vi "kinectConfigure.vi"(8 "error in (no error)":errorcluster, 10 "Enabled Frames":T2, 11 "KinectSensor References in":T1) -> (0 "error out":errorcluster, 3 "KinectSensor References out":T1)   [LabVIEW 2014]
uses:
  controls/KinectSensor References.ctl
  Microsoft.Kinect
  controls/FrameDescription.ctl
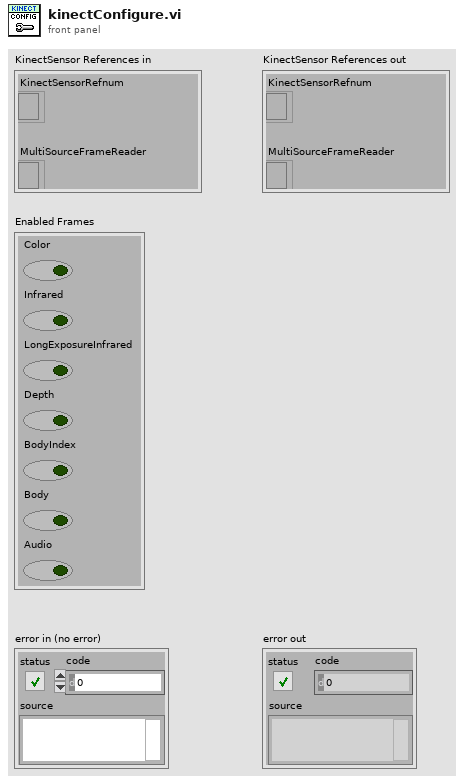
[diagram p1: front panel]
types:
  T1 = typedef "KinectSensor References.ctl" = cluster{"KinectSensorRefnum":refnum<k24>, "MultiSourceFrameReader":refnum<k24>}
  T2 = cluster{"Color":bool, "Infrared":bool, "LongExposureInfrared":bool, "Depth":bool, "BodyIndex":bool, "Body":bool, "Audio":bool}
  T3 = typedef "FrameDescription.ctl" = cluster{"BytesPerPixel":u32, "DiagonalFieldOfView":sgl, "Height":i32, "HorizontalFieldOfView":sgl, "LengthInPixels":u32, "VerticalFieldOfView":sgl, "Width":i32}
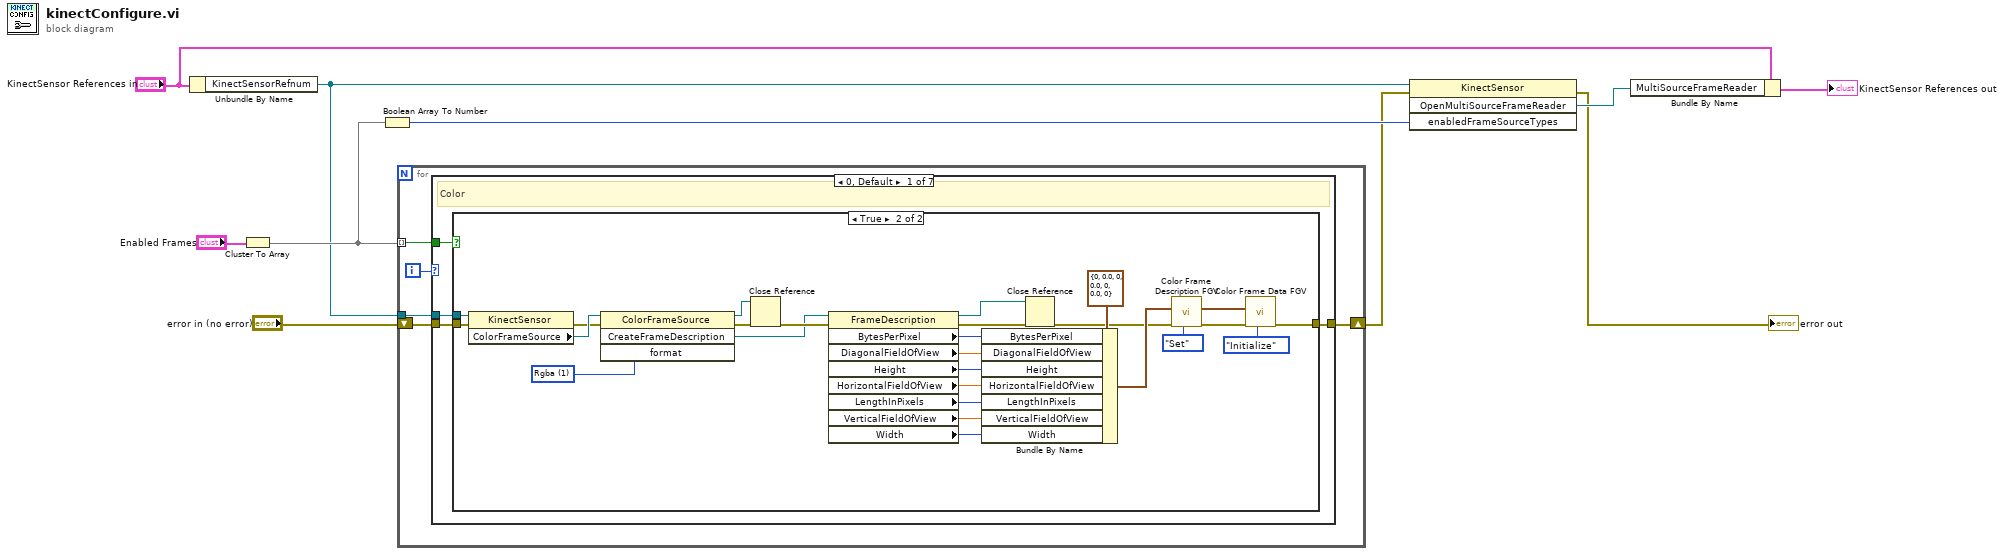
[diagram p0: block diagram]
diagram:
  n1 = Unbundle By Name("KinectSensor References in") -> ("KinectSensorRefnum"=w3:refnum<k24>)
  n2 = Cluster To Array(cluster="Enabled Frames") -> (array=w9:bool[])
  n3 = Boolean Array To Number(Boolean array=w9) -> (number=w5:u32)
  n4 = for {
    tunnel: w9 -> [w14] mode=indexing
    shift-right: [w12] -> w2
    shift-left: "error in (no error)" -> [w13]
    tunnel: w3 -> [w11]
    i -> [w15]
    n5 = case shown="0, Default" w15 {
      tunnel: w14 -> [w19 _ _ _ _ _ _]
      tunnel: w13 -> [w18 w47 w48 w49 w50 w51 w52]
      tunnel: [w17 w47 w48 w49 w50 w51 w52] -> w12
      tunnel: w11 -> [w16 _ _ _ _ _ _]
      frame 0, Default {
        # "Color"
        n6 = case shown="True" w19 {
          tunnel: w18 -> [w20 w34]
          tunnel: [w20 w33] -> w17
          tunnel: w16 -> [_ w27]
          frame False {
          }
          frame True {
            w21 = 1 items=["None", "Rgba", "Yuv", "Bgra", "Bayer", "Yuy2"] ("format")
            n7 = property class="KinectSensor"(reference=w27, error in=w34) -> (error out=w22:errorcluster, "ColorFrameSource"=w25:refnum<k24>)  [unwired: 1 out]
            n8 = invoke class="ColorFrameSource" method="CreateFrameDescription"(reference=w25, error in=w22, "format"=w21) -> (reference out=w23:refnum<k24>, error out=w26:errorcluster, "CreateFrameDescription"=w24:refnum<k24>)  [unwired: 1 in, 1 out]
            n9 = Close Reference(reference=w23, error in (no error)=w26) -> (error out=w30:errorcluster)
            n10 = property class="FrameDescription"(reference=w24, error in=w30) -> (reference out=w31:refnum<k24>, error out=w32:errorcluster, "BytesPerPixel"=w36:u32, "DiagonalFieldOfView"=w37:sgl, "Height"=w38:i32, "HorizontalFieldOfView"=w39:sgl, "LengthInPixels"=w40:u32, "VerticalFieldOfView"=w41:sgl, "Width"=w42:i32)
            n11 = Bundle By Name(cluster=T3 {"BytesPerPixel"=0, "DiagonalFieldOfView"=0.0, "Height"=0, "HorizontalFieldOfView"=0.0, "LengthInPixels"=0, "VerticalFieldOfView"=0.0, "Width"=0} ("FrameDescription"), "BytesPerPixel"=w36, "DiagonalFieldOfView"=w37, "Height"=w38, "HorizontalFieldOfView"=w39, "LengthInPixels"=w40, "VerticalFieldOfView"=w41, "Width"=w42) -> (w43:T3)
            n12 = Close Reference(reference=w31, error in (no error)=w32) -> (error out=w29:errorcluster)
            n13 = call "Color Frame Description FGV.vi"("Command"=enum16{"Get", "Set"}."Set", "error in (no error)"=w29, "FrameDescription"=w43) -> ("error out"=w46:errorcluster, "FrameDescription"=w28:T3)  [unwired: 7 in]
            n14 = call "Color Frame Data FGV.vi"("Command"=enum16{"Get", "Initialize"}."Initialize", "error in (no error)"=w46, "FrameDescription"=w28) -> ("error out"=w33:errorcluster)  [unwired: 7 in, 1 out]
          }
        }
      }
      frame 1 {
        # "Infrared"
      }
      frame 2 {
        # "LongExposureInfrared"
      }
      frame 3 {
        # "Depth"
      }
      frame 4 {
        # "BodyIndex"
      }
      frame 5 {
        # "Body"
      }
      frame 6 {
        # "Audio"
      }
    }
  }
  n15 = invoke class="KinectSensor" method="OpenMultiSourceFrameReader"(reference=w3, error in=w2, "enabledFrameSourceTypes"=w5) -> (error out=→"error out":errorcluster, "OpenMultiSourceFrameReader"=w7:refnum<k24>)  [unwired: 1 in, 2 out]
  n16 = Bundle By Name(cluster="KinectSensor References in", "MultiSourceFrameReader"=w7) -> (→"KinectSensor References out":T1)
